vi "Eval_MultiVar_BulkMode.vi"(8 "error in (no error)":errorcluster, 9 "varValues":dbl[][](array[numeric]) format="%#_13g", 10 "varNames":string[](array[string]), 11 "mupExpr in":refnum<data-value>) -> (0 "error out":errorcluster, 2 "Result":dbl[](array[numeric]) format="%#_13g", 3 "mupExpr out":refnum<data-value>)   [LabVIEW 2015, in "mupExpr.lvclass"]
doc: "Update the value of multiple variables then evaluate the expression in bulk mode. Returns the array of results.\n\nNote that the array of values provided for variable values should be of size:\nNum Rows: Number of Variables\nNum Cols: Bulk Size\n\nIf any variable is not found, a warning is generated.\n\nIf multiple expressions have been input, the last one in the list is evaluated."
uses:
  mupExpr.lvclass
  mupExpr.lvclass/mupExpr.ctl
  mupLib/mupSetVarValue_Array.vi
  mupLib/mupCheckError.vi
  mupLib/mupLibPath.vi
  <vilib>/Utility/error.llb/Error Cluster From Error Code.vi
  mupLib/mupLib.lvlib
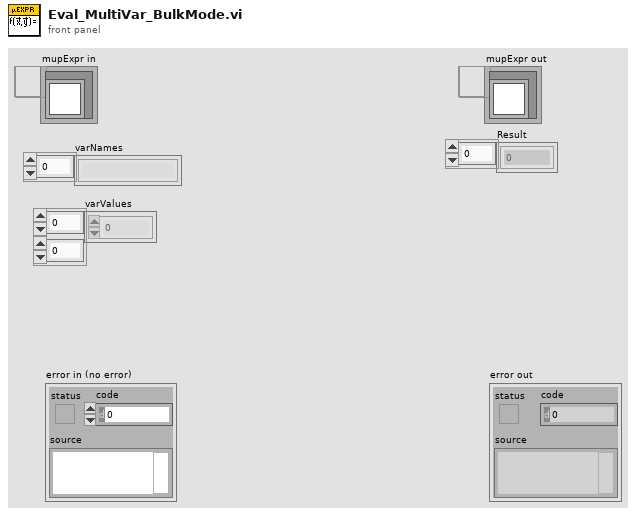
[diagram p1: front panel]
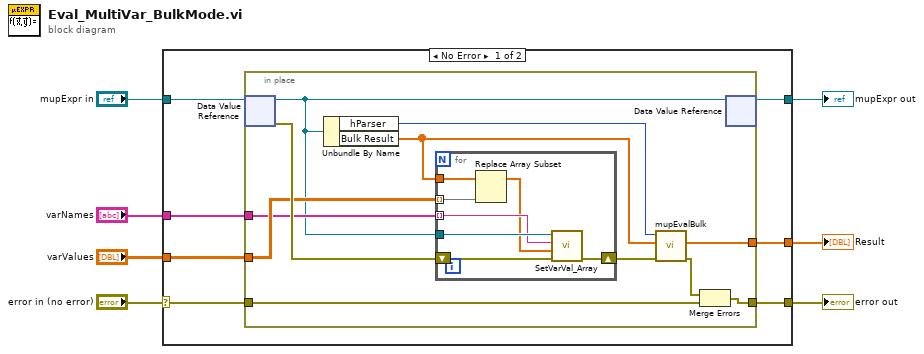
[diagram p0: block diagram]
diagram:
  n1 = case shown="No Error" "error in (no error)" {
    selector: "error in (no error)" -> [w9 w34]
    tunnel: "varValues" -> [w14 _]
    tunnel: "varNames" -> [w13 _]
    tunnel: [w12 _] -> w6
    tunnel: "mupExpr in" -> [w11 w33]
    tunnel: [w8 w34] -> w4
    tunnel: [w10 w33] -> w3
    frame No Error {
      n2 = in-place {
        in-place-border: w9 -> [w17]
        in-place-border: [w20] -> w12
        in-place-border: w14 -> [w24]
        in-place-border: w13 -> [w23]
        in-place-border: [w15] -> w8
        n3 = in-place-dvr #1(w11) -> (w18:refnum<class "mupExpr.lvclass">, w25:errorcluster)
        n4 = Unbundle By Name(w18) -> ("hParser"=w21:u64, "Bulk Result"=w22:dbl[])
        n5 = for {
          tunnel: w23 -> [w28] mode=indexing
          tunnel: w24 -> [w27] mode=indexing
          shift-right: [w30] -> w19
          shift-left: w25 -> [w31]
          tunnel: w22 -> [w32]
          tunnel: w18 -> [w29]
          n6 = Replace Array Subset(array=w32, new element=w27) -> (w26:dbl[])  [unwired: 1 in]
          n7 = call "SetVarVal_Array.vi"("error in (no error)"=w31, "varValue"=w26, "varName"=w28, "muExpr in"=w29) -> ("error out"=w30:errorcluster)  [unwired: 6 in, 1 out]
        }
        n8 = call "mupEvalBulk.vi"("error in (no error)"=w19, "a_res"=w22, "hParser in"=w21) -> ("error out"=w16:errorcluster, "results"=w20:dbl[])  [unwired: 6 in, 1 out]
        n9 = Merge Errors(w16, w17) -> (w15:errorcluster)
        n10 = in-place-dvr #1(w18) -> (w10:refnum<data-value>)  [unwired: 1 out]
      }
    }
    frame Error {
    }
  }
  "error out" <- w4
  "mupExpr out" <- w3
  "Result" <- w6
